vi "x and y subarray 2.vi"(8 "Turn on itself":bool, 10 "Encoder  Right":dbl[](array[numeric]), 11 "Encoder Left":dbl[](array[numeric])) -> (0 "Heading":dbl, 2 "x":dbl, 3 "y":dbl)   [LabVIEW 2013]
panel:
  in  "y Starting position":dbl format="%#_13g"
  in  "x Starting position":dbl format="%#_13g"
  in  "distance between wheels":dbl=110.0
  out "Sr":dbl
  out "Sl":dbl
  in  "wheel circumference":dbl=132.0
  in  "Resolution":dbl=48.0 format="%#_13g"
  # "Bot dimensions\nand other things that \nwe have to initialize"
  # "Inputs"
  # "Useless"
  # "Outputs"
  # "Correct distances:\n132\n124"
  # "but try 132\n110"
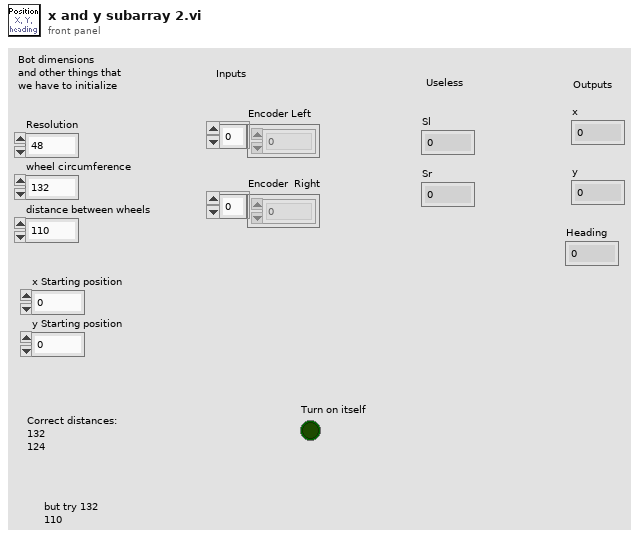
[diagram p1: front panel]
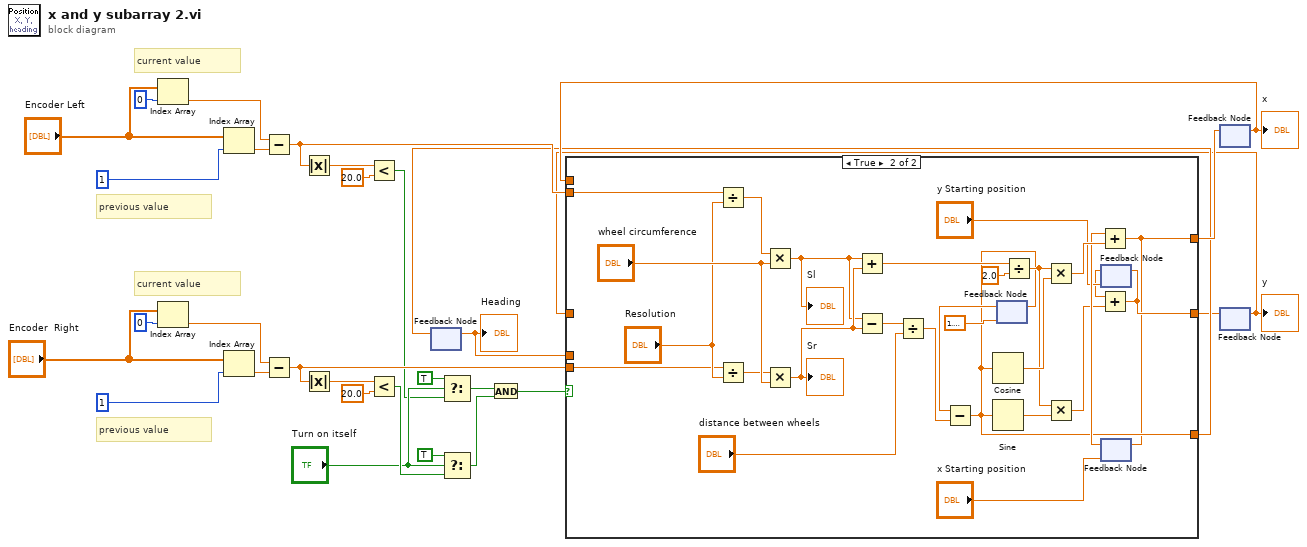
[diagram p0: block diagram]
diagram:
  # "previous value"
  # "current value"
  # "previous value"
  # "current value"
  n1 = Index Array(array="Encoder Left", index=0) -> (element=w29:dbl)
  n2 = Index Array(array="Encoder  Right", index=0) -> (element=w26:dbl)
  n3 = Index Array(array="Encoder Left", index=1) -> (element=w28:dbl)
  n4 = Index Array(array="Encoder  Right", index=1) -> (element=w27:dbl)
  n5 = Subtract(x=w29, y=w28) -> (x-y=w20:dbl)
  n6 = Subtract(x=w26, y=w27) -> (x-y=w19:dbl)
  n7 = Absolute Value(x=w20) -> (abs(x)=w16:dbl)
  n8 = Absolute Value(x=w19) -> (abs(x)=w15:dbl)
  n9 = Less?(x=w16, y=20.0) -> (x < y?=w2:bool)
  n10 = Less?(x=w15, y=20.0) -> (x < y?=w6:bool)
  n11 = feedback #1() -> (w10:dbl)  [unwired: 1 in]
  "Heading" <- w10
  n12 = Select(t=TRUE, s="Turn on itself", f=w2) -> (s? t:f=w1:bool)
  n13 = Select(t=TRUE, s="Turn on itself", f=w6) -> (s? t:f=w5:bool)
  n14 = And(x=w1, y=w5) -> (x .and. y?=w14:bool)
  n15 = feedback #2() -> (w12:dbl)  [unwired: 1 in]
  "x" <- w12
  n16 = feedback #3() -> (w8:dbl)  [unwired: 1 in]
  "y" <- w8
  n17 = case shown="True" w14 {
    tunnel: w20 -> [_ w41]
    tunnel: w19 -> [_ w40]
    tunnel: [w32 w36] -> w11
    tunnel: [w31 w35] -> w9
    tunnel: [w33 w34] -> w13
    tunnel: w12 -> [w33 _]
    tunnel: w10 -> [w32 _]
    tunnel: w8 -> [w31 _]
    frame False {
    }
    frame True {
      n18 = Divide(x=w41, y="Resolution") -> (x/y=w42:dbl)
      n19 = Divide(x=w40, y="Resolution") -> (x/y=w43:dbl)
      n20 = Multiply(x=w42, y="wheel circumference") -> (x*y=w50:dbl)
      "Sl" <- w50
      n21 = Multiply(x=w43, y="wheel circumference") -> (x*y=w51:dbl)
      "Sr" <- w51
      n22 = Add(x=w50, y=w51) -> (x+y=w38:dbl)
      n23 = Subtract(x=w50, y=w51) -> (x-y=w46:dbl)
      n24 = Divide(x=w46, y="distance between wheels") -> (x/y=w48:dbl)
      n25 = feedback #4(1.5707963267948966) -> (w49:dbl)
      n26 = Subtract(x=w49, y=w48) -> (x-y=w36:dbl)
      n27 = Cosine(x=w36) -> (cos(x)=w56:dbl)
      n28 = Sine(x=w36) -> (sin(x)=w52:dbl)
      n29 = feedback-in #4(w36) -> ()
      n30 = Divide(x=w38, y=2.0) -> (x/y=w37:dbl)
      n31 = Multiply(x=w37, y=w56) -> (x*y=w59:dbl)
      n32 = Multiply(x=w37, y=w52) -> (x*y=w53:dbl)
      n33 = feedback #5("y Starting position") -> (w54:dbl)
      n34 = Add(x=w54, y=w53) -> (x+y=w35:dbl)
      n35 = feedback-in #5(w35) -> ()
      n36 = feedback #6("x Starting position") -> (w57:dbl)
      n37 = Add(x=w57, y=w59) -> (x+y=w34:dbl)
      n38 = feedback-in #6(w34) -> ()
    }
  }
  n39 = feedback-in #1(w11) -> ()
  n40 = feedback-in #2(w13) -> ()
  n41 = feedback-in #3(w9) -> ()
